vi "Connection Get Data.vi"(8 "error in (no error)":errorcluster, 10 "Expression in":string, 11 "Connection DVR in":refnum<data-value>) -> (0 "error out":errorcluster, 2 "Data DVR out":refnum<data-value>, 3 "Connection DVR out":refnum<data-value>)   [LabVIEW 2012, in "MDSplus.lvlib"]
uses:
  <vilib>/MDSplus/Library/MDSplus.lvlib
  <vilib>/MDSplus/Classes/Connection_Class/Connection.lvclass
  <vilib>/MDSplus/Classes/Data_Class/Data.lvclass
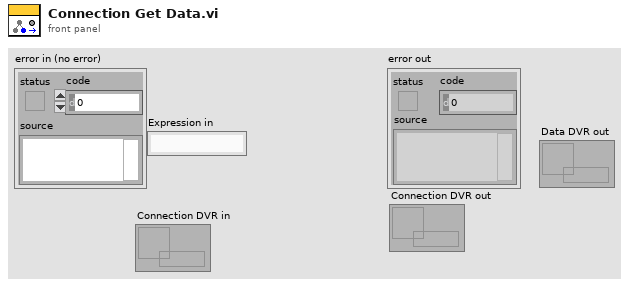
[diagram p1: front panel]
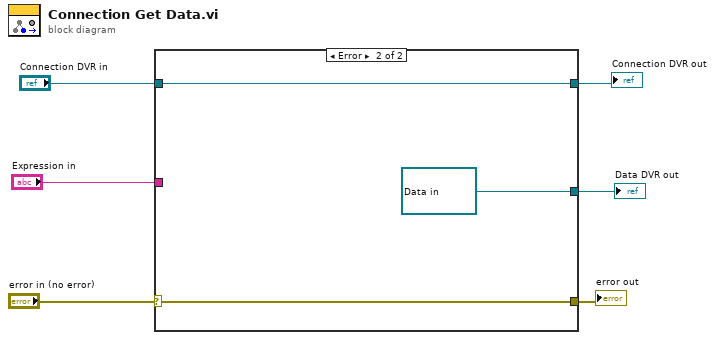
[diagram p0: block diagram]
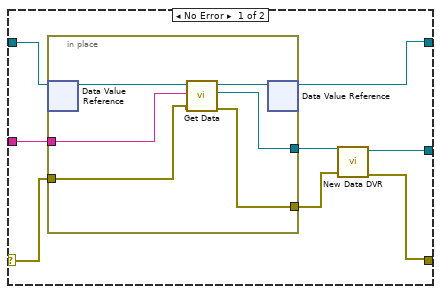
[diagram p2: hidden frame]
diagram:
  n1 = case shown="Error" "error in (no error)" {
    selector: "error in (no error)" -> [w11 w23]
    tunnel: [w7 w23] -> w5
    tunnel: "Connection DVR in" -> [w14 w22]
    tunnel: [w13 w22] -> w3
    tunnel: "Expression in" -> [w12 _]
    tunnel: [w9 refnum<data-value> refnum ("Data DVR out 2")] -> w1
    frame No Error {
      n2 = in-place {
        in-place-border: w12 -> [w18]
        in-place-border: w11 -> [w17]
        in-place-border: [w16] -> w8
        in-place-border: [w15] -> w10
        n3 = in-place-dvr #1(w14) -> (w20:refnum<class "Connection.lvclass">)  [unwired: 1 out]
        n4 = call <vilib>:"Get Data.vi"("error in (no error)"=w17, "Expression in"=w18, "Connection in"=w20) -> ("error out"=w16:errorcluster, "Data out"=w15:refnum<class "Data.lvclass">, "Connection out"=w19:refnum<class "Connection.lvclass">)  [unwired: 6 in]
        n5 = in-place-dvr #1(w19) -> (w13:refnum<data-value>)  [unwired: 1 out]
      }
      n6 = call <vilib>:"New Data DVR.vi"("error in (no error)"=w8, "Data in"=w10) -> ("error out"=w7:errorcluster, "Data DVR out"=w9:refnum<data-value>)  [unwired: 8 in]
    }
    frame Error {
    }
  }
  "error out" <- w5
  "Connection DVR out" <- w3
  "Data DVR out" <- w1
